vi "Read Abberation from Excel.vi"(9 "Ring":u16(ring)) -> (2 "output cluster":T1)   [LabVIEW 2014]
doc: "This example opens a worksheet in a specified Excel workbook and extracts data from the spreadsheet. The data can be interpreted either as numeric or string data, and the data can be in the form of a single cell of data or a 2D array.\n\nSelect an Excel workbook with the path control, specify a range of cells to read. Then go to\nthe block diagram and select the polymorphic instance corresponding to the type and range of data to read. You might have to recreate an indicator for the data if you change instances. Press run to extract the data from the Excel workbook."
uses:
  AbberationControl.ctl
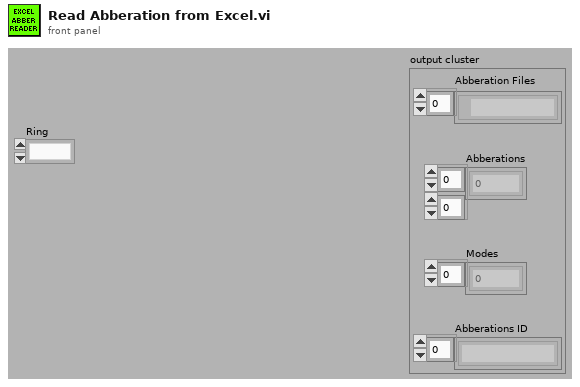
[diagram p1: front panel]
types:
  T1 = typedef "AbberationControl.ctl" = cluster{"Abberations":dbl[][], "Modes":i32[], "Abberations ID":string[], "Abberation Files":path[]}
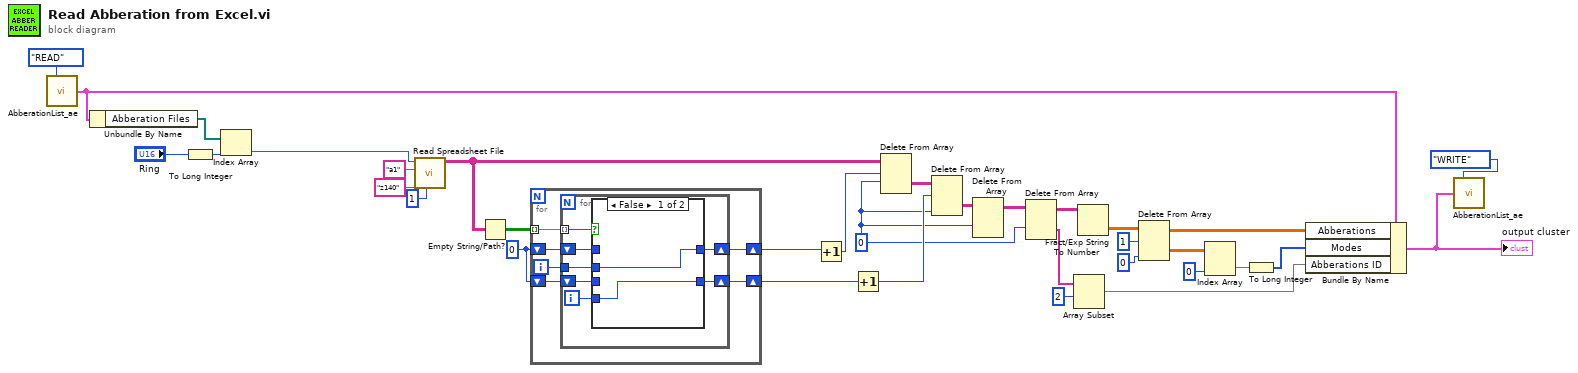
[diagram p0: block diagram]
diagram:
  w24 = 0 ("disabled index (col)")
  w25 = 0
  n1 = call "AbberationList_ae.vi"("Enum"=enum16{"WRITE", "READ"}."READ") -> ("Abberation Cluster Out"=w3:T1)  [unwired: 14 in]
  n2 = Unbundle By Name(w3) -> ("Abberation Files"=w4:path[])
  n3 = To Long Integer(number="Ring") -> (32bit integer=w7:i32)
  n4 = Index Array(array=w4, index=w7) -> (element=w6:path)
  n5 = call "Read Spreadsheet File.vi"("Sheet No"=1, "End cell"="z140", "Start Cell"="a1", "path"=w6) -> ("Array"=w10:string[][])  [unwired: 6 in, 1 out]
  n6 = Empty String/Path?(string/path=w10) -> (empty?=w34:bool[][])
  n7 = for {
    tunnel: w34 -> [w40] mode=indexing
    shift-right: [w39] -> w32
    shift-left: w25 -> [w36]
    shift-right: [w38] -> w31
    shift-left: w25 -> [w35]
    i -> [w37]
    n8 = for {
      tunnel: w40 -> [w47] mode=indexing
      shift-right: [w44] -> w39
      shift-left: w36 -> [w46]
      shift-right: [w43] -> w38
      shift-left: w35 -> [w42]
      tunnel: w37 -> [w41]
      i -> [w45]
      n9 = case shown="False" w47 {
        tunnel: w46 -> [_ w50]
        tunnel: w45 -> [w49 _]
        tunnel: [w48 w50] -> w44
        tunnel: [w49 w51] -> w43
        tunnel: w42 -> [_ w51]
        tunnel: w41 -> [w48 _]
        frame False {
        }
        frame True {
        }
      }
    }
  }
  n10 = Increment(x=w32) -> (x+1=w30:i32)
  n11 = Increment(x=w31) -> (x+1=w29:i32)
  n12 = Delete From Array(array=w10, length=w30, index (row)=w24) -> (deleted portion=w33:string[][])  [unwired: 1 in, 1 out]
  n13 = Delete From Array(array=w33, length=w29, index (col)=w24) -> (deleted portion=w28:string[][])  [unwired: 1 in, 1 out]
  n14 = Delete From Array(array=w28, index (row)=w24) -> (array with subset deleted=w27:string[][])  [unwired: 2 in, 1 out]
  n15 = Delete From Array(array=w27, index (row)=w24) -> (deleted portion=w23:string[], array with subset deleted=w26:string[][])  [unwired: 2 in]
  n16 = Array Subset(array=w23, index=2 ("length")) -> (w9:string[])  [unwired: 1 in]
  n17 = Fract/Exp String To Number(string=w26) -> (number=w21:dbl[][])  [unwired: 3 in, 1 out]
  n18 = Delete From Array(array=w21, length=1, index (col)=0 ("disabled index (col)")) -> (deleted portion=w18:dbl[][], array with subset deleted=w15:dbl[][])  [unwired: 1 in]
  n19 = Index Array(array=w18, index (col)=0 ("disabled index (col)")) -> (element=w16:dbl[])  [unwired: 1 in]
  n20 = To Long Integer(number=w16) -> (32bit integer=w14:i32[])
  n21 = Bundle By Name(cluster=w3, "Abberations"=w15, "Modes"=w14, "Abberations ID"=w9) -> (w1:T1)
  "output cluster" <- w1
  n22 = call "AbberationList_ae.vi"("Enum"=enum16{"WRITE", "READ"}."WRITE", "Abberation Cluster In"=w1) -> ()  [unwired: 13 in, 1 out]
